vi "Begin Initialization.vi"   [LabVIEW 2016]
uses:
  <vilib>/Rock Robotics/WPI/DriverStation/WPI_DriverStationRobotMode2.ctl
  <vilib>/Rock Robotics/WPI/Joystick/WPI_JoystickDeviceEnum.ctl
  <vilib>/Rock Robotics/WPI/ThirdParty/CanMotor/TalonSRX/WPI_CANTalonSRX_APIControlMode.ctl
  <vilib>/Rock Robotics/WPI/Solenoid/WPI_SolenoidChannel.ctl
  <vilib>/Rock Robotics/SystemInterfaces/DIO/FPGA_DIOChannel.ctl
  <vilib>/Rock Robotics/WPI/ThirdParty/CanMotor/TalonSRX/WPI_CANTalonSRX_APIFeedbackSelect.ctl
  <vilib>/Rock Robotics/WPI/Solenoid/WPI_SolenoidValue.ctl
  <vilib>/Rock Robotics/SystemInterfaces/DIO/FPGA_DIOPWMChannel.ctl
  Robot Global Data.vi
  <vilib>/Rock Robotics/WPI/Solenoid/WPI_SolenoidOpenDouble.vi
  Global Variables/Robot Status.vi
  <vilib>/Rock Robotics/WPI/MotorControl/WPI_MotorControlOpen Talon.vi
  Global Variables/Refnum Names.vi
  <vilib>/Rock Robotics/WPI/ThirdParty/Sensors/Pigeon IMU/CTRE_PigeonIMU_Open_TalonSRX.vi
  <vilib>/Rock Robotics/WPI/Solenoid/WPI_SolenoidSetEnum.vi
  Global Variables/Folder Names.vi
  Global Variables/MotionProfile.vi
  Global Variables/Low Gear Calibrations.vi
  Global Variables/High Gear Calibrations.vi
types:
  T1 = typedef "WPI_CANTalonSRX_APIControlMode.ctl" = enum8{"Percent VBus", "Speed", "Position", "Slave", "Unchanged / Invalid", "Voltage Compensation", "Current", "Motion Profile", "Motion Magic"}
  T2 = typedef "FPGA_DIOChannel.ctl" = enum8{"DIO 0", "DIO 1", "DIO 2", "DIO 3", "DIO 4", "DIO 5", "DIO 6", "DIO 7", "DIO 8", "DIO 9", "DIO MXP 0", "DIO MXP 1", "DIO MXP 2", "DIO MXP 3", "DIO MXP 4", "DIO MXP 5", "DIO MXP 6", "DIO MXP 7", "DIO MXP 8", "DIO MXP 9", "DIO MXP 10", "DIO MXP 11", "DIO MXP 12", "DIO MXP 13", "DIO MXP 14", "DIO MXP 15", "SPI Port CS1", "SPI Port CS2", "SPI Port CS3", "SPI Port MISO", "SPI Port MOSI", "Invalid"}
  T3 = typedef "WPI_SolenoidValue.ctl" = enum16{"Off", "On", "Forward", "Reverse"}
  T4 = typedef "WPI_SolenoidChannel.ctl" = enum8{"Solenoid 0", "Solenoid 1", "Solenoid 2", "Solenoid 3", "Solenoid 4", "Solenoid 5", "Solenoid 6", "Solenoid 7", "Invalid"}
  T5 = typedef "FPGA_DIOPWMChannel.ctl" = enum8{"PWM 0", "PWM 1", "PWM 2", "PWM 3", "PWM 4", "PWM 5", "PWM 6", "PWM 7", "PWM 8", "PWM 9", "PWM MXP 0", "PWM MXP 1", "PWM MXP 2", "PWM MXP 3", "PWM MXP 4", "PWM MXP 5", "PWM MXP 6", "PWM MXP 7", "PWM MXP 8", "PWM MXP 9", "Invalid"}
  T6 = typedef "WPI_JoystickDeviceEnum.ctl" = enum16{"USB 0", "USB 1", "USB 2", "USB 3", "USB 4", "USB 5"}
  T7 = typedef "WPI_CANTalonSRX_APIFeedbackSelect.ctl" = enum16{"Digital Quadrature Encoder", "Analog Potentiometer", "Analog Encoder", "Count on Quad-A (Rising-Edge)", "Count on Quad-A (Falling-Edge)", "CTR Magnetic Enc (Absolute)", "CTR Magnetic Enc (Relative)", "Pulse Width"}
  T8 = typedef "WPI_DriverStationRobotMode2.ctl" = enum16{"Autonomous Disabled", "Autonomous Enabled", "Teleop Disabled", "Teleop Enabled", "Disconnected", "Finish", "Test Disabled", "Test Enabled", "Emergency Stopped"}
  T9 = typedef "WPI_JoystickDevRef.ctl" = cluster{"Device":T6}
  T10 = typedef "WPI_MotorControlDeviceRef.ctl" = cluster{"DeviceStatus":errorcluster, "Type":T11, "PWM":cluster{"PWM Channel":T5, "DeadBand":T12}, "CAN":cluster{"Device Number":u8, "SetOutput VI Ref":variant, "GetOutput VI Ref":variant, "Enable VI Ref":variant, "Disable VI Ref":variant, "Data":variant}, "Invert":bool}
  T11 = typedef "WPI_MotorControlType.ctl" = enum16{"PWM", "CAN"}
  T12 = typedef "WPI_PWMDeadband.ctl" = cluster{"Name":string, "maxPositivePwm":i32, "minPositivePwm":i32, "centerPwm":i32, "maxNegativePwm":i32, "minNegativePwm":i32, "angularRange":u16}
  T13 = typedef "MotionProfile TypeDef.ctl" = cluster{"Left MP Array":dbl[][], "Left MP Index":dbl, "Semaphore":bool, "Right MP Array":dbl[][], "Right MP Index":dbl}
  T14 = typedef "CTRE_PigeonIMU_DeviceRef.ctl" = cluster{"DeviceStatus":errorcluster, "Device Number":u8, "Type":T15, "Device ID":u32}
  T15 = typedef "CTRE_PigeonIMU_ConnectionType.ctl" = u32
  T16 = typedef "WPI_SolenoidDevRef.ctl" = cluster{"DevStatus":errorcluster, "Pneumatics Control Module":u8, "Forward Solenoid Channel":T4, "Reverse Solenoid Channel":T4}
  T17 = typedef "WPI_DigitalOutputDevRef.ctl" = cluster{"DIO Channel":T2, "DevStatus":errorcluster}
  T18 = typedef "WPI_DigitalInputDevRef.ctl" = cluster{"DevStatus":errorcluster, "DIO Channel":T2}
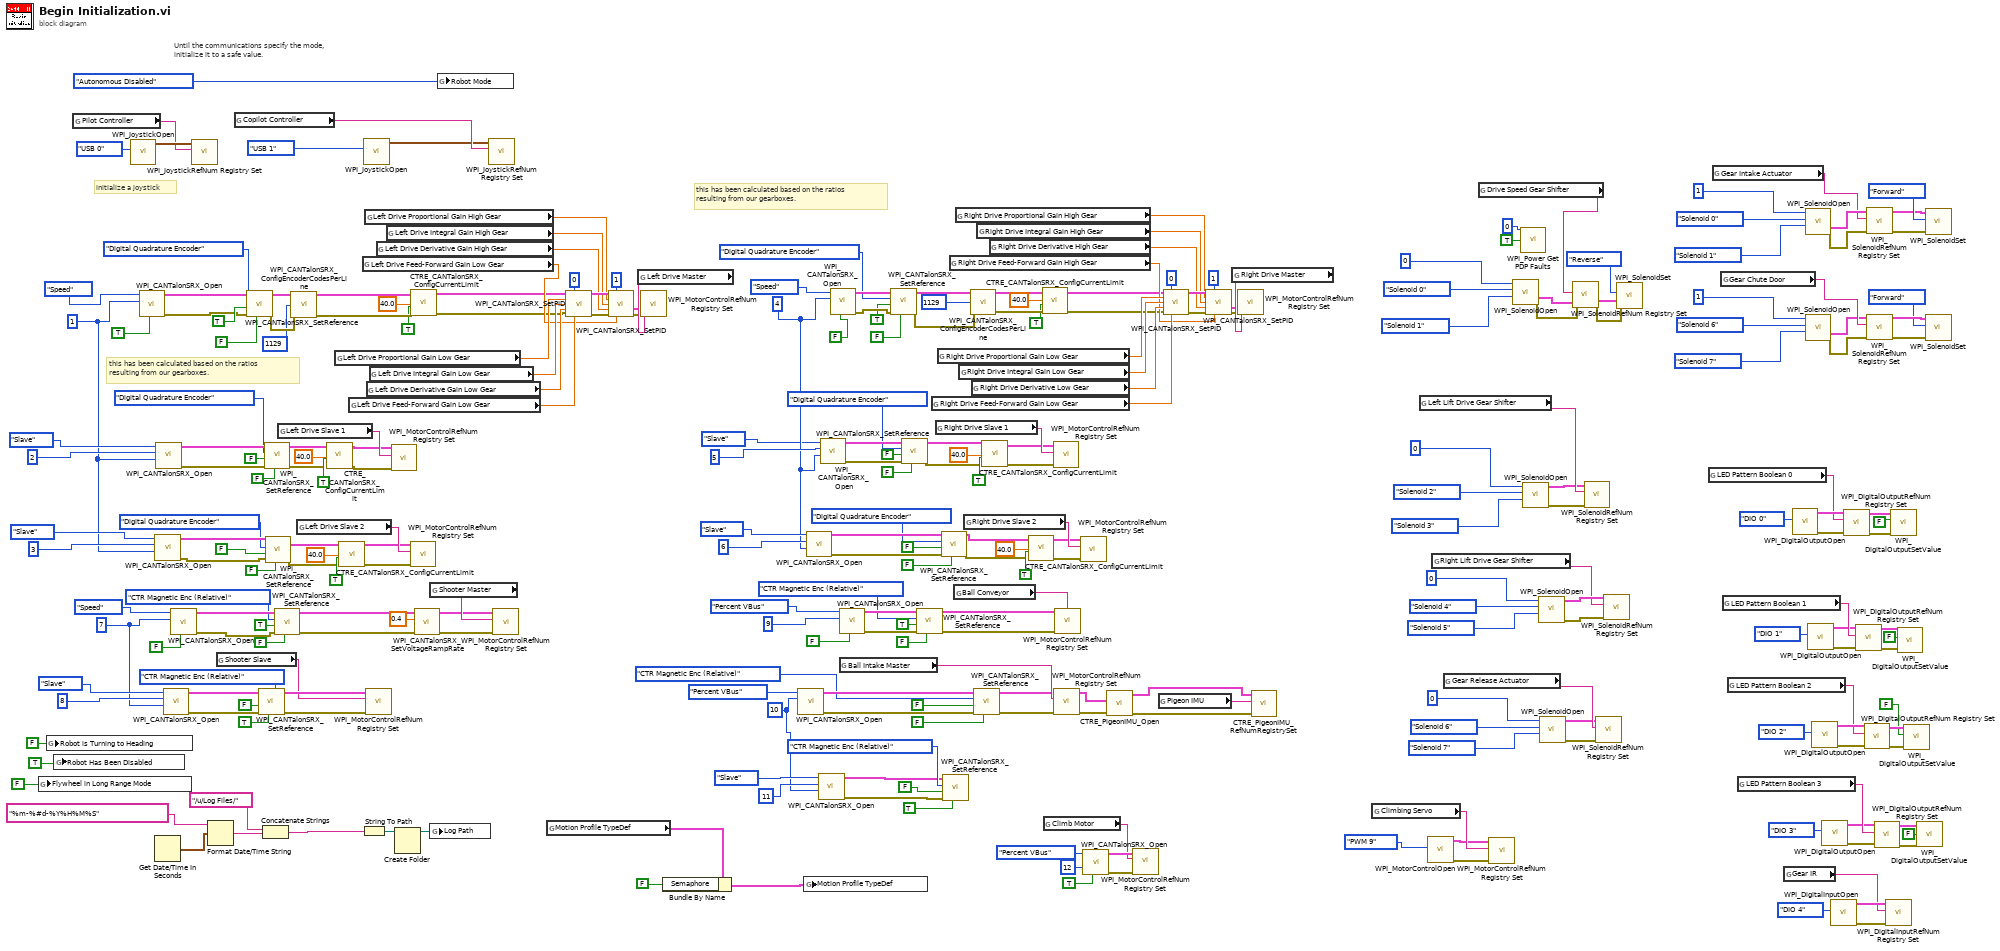
[diagram p0: block diagram]
diagram:
  w155 = u8 10 ("Device Number")
  w259 = u8 7 ("Device Number")
  w258 = u8 4 ("Device Number")
  w260 = u8 1 ("Device Number")
  # "this has been calculated based on the ratios\nresulting from our gearboxes."
  # "this has been calculated based on the ratios\nresulting from our gearboxes."
  # "initialize a joystick"
  # "Until the communications specify the mode,\ninitialize it to a safe value."
  n1 = global write "Robot Status.vi" "Flywheel in Long Range Mode"(FALSE) -> ()
  n2 = global write "Robot Status.vi" "Robot is Turning to Heading"(FALSE ("Robot is Turning to Heading")) -> ()
  n3 = global write "Robot Status.vi" "Robot Has Been Disabled"(TRUE) -> ()
  n4 = global read "Refnum Names.vi" "Pilot Controller"() -> (w248:string)
  n5 = call <vilib>:"WPI_JoystickOpen.vi"("JoystickDevice"=WPI_JoystickDeviceEnum."USB 0") -> ("JoystickDevRef"=w283:T9)  [unwired: 10 in]
  n6 = call <vilib>:"WPI_CANTalonSRX_Open.vi"("Invert"=TRUE, "Device Number"=w260, "Control Mode"=WPI_CANTalonSRX_APIControlMode."Speed") -> ("error out"=w195:errorcluster, "CAN Talon SRX Ref"=w280:T10)  [unwired: 7 in]
  n7 = call <vilib>:"WPI_CANTalonSRX_Open.vi"("Master Device Number"=w260, "Device Number"=u8 3, "Control Mode"=WPI_CANTalonSRX_APIControlMode."Slave") -> ("error out"=w193:errorcluster, "CAN Talon SRX Ref"=w273:T10)  [unwired: 7 in]
  n8 = Get Date/Time In Seconds() -> (seconds since 1Jan1904=w137:timestamp)
  n9 = call <vilib>:"WPI_CANTalonSRX_Open.vi"("Master Device Number"=w260, "Device Number"=u8 2, "Control Mode"=WPI_CANTalonSRX_APIControlMode."Slave") -> ("error out"=w194:errorcluster, "CAN Talon SRX Ref"=w278:T10)  [unwired: 7 in]
  n10 = call <vilib>:"WPI_CANTalonSRX_Open.vi"("Master Device Number"=w259, "Device Number"=u8 8, "Control Mode"=WPI_CANTalonSRX_APIControlMode."Slave") -> ("error out"=w187:errorcluster, "CAN Talon SRX Ref"=w261:T10)  [unwired: 7 in]
  n11 = call <vilib>:"WPI_CANTalonSRX_Open.vi"("Invert"=FALSE, "Device Number"=w259, "Control Mode"=WPI_CANTalonSRX_APIControlMode."Speed") -> ("error out"=w189:errorcluster, "CAN Talon SRX Ref"=w265:T10)  [unwired: 7 in]
  n12 = call <vilib>:"WPI_JoystickRefNum Registry Set.vi"("refnum name"=w248, "JoystickDevRef"=w283) -> ()  [unwired: 8 in, 2 out]
  n13 = Format Date/Time String(time format string (%c)="%m-%#d-%Y%H%M%S", seconds (now)=w137) -> (date/time string=w135:string)  [unwired: 1 in]
  n14 = global read "Refnum Names.vi" "Shooter Slave"() -> (w123:string)
  n15 = global read "Refnum Names.vi" "Copilot Controller"() -> (w153:string)
  n16 = call <vilib>:"WPI_CANTalonSRX_SetReference.vi"("Reverse Closed-Loop Output"=FALSE, "error in (no error)"=w195, "Reverse Feedback Sensor"=TRUE, "Feedback Reference"=WPI_CANTalonSRX_APIFeedbackSelect."Digital Quadrature Encoder", "CAN Talon SRX Ref"=w280) -> ("error out"=w150:errorcluster, "CAN Talon SRX Ref"=w204:T10)  [unwired: 5 in]
  n17 = call <vilib>:"WPI_CANTalonSRX_SetReference.vi"("Reverse Closed-Loop Output"=TRUE, "error in (no error)"=w187, "Reverse Feedback Sensor"=FALSE, "Feedback Reference"=WPI_CANTalonSRX_APIFeedbackSelect."CTR Magnetic Enc (Relative)", "CAN Talon SRX Ref"=w261) -> ("error out"=w125:errorcluster, "CAN Talon SRX Ref"=w124:T10)  [unwired: 5 in]
  n18 = Concatenate Strings("/u/Log Files/" ("string"), w135) -> (w133:string)
  n19 = call <vilib>:"WPI_CANTalonSRX_SetReference.vi"("Reverse Closed-Loop Output"=FALSE, "error in (no error)"=w194, "Reverse Feedback Sensor"=FALSE, "Feedback Reference"=WPI_CANTalonSRX_APIFeedbackSelect."Digital Quadrature Encoder", "CAN Talon SRX Ref"=w278) -> ("error out"=w19:errorcluster, "CAN Talon SRX Ref"=w20:T10)  [unwired: 5 in]
  n20 = call <vilib>:"WPI_CANTalonSRX_SetReference.vi"("Reverse Closed-Loop Output"=FALSE, "error in (no error)"=w193, "Reverse Feedback Sensor"=FALSE, "Feedback Reference"=WPI_CANTalonSRX_APIFeedbackSelect."Digital Quadrature Encoder", "CAN Talon SRX Ref"=w273) -> ("error out"=w14:errorcluster, "CAN Talon SRX Ref"=w15:T10)  [unwired: 5 in]
  n21 = call <vilib>:"WPI_CANTalonSRX_SetReference.vi"("Reverse Closed-Loop Output"=FALSE, "error in (no error)"=w189, "Reverse Feedback Sensor"=TRUE, "Feedback Reference"=WPI_CANTalonSRX_APIFeedbackSelect."CTR Magnetic Enc (Relative)", "CAN Talon SRX Ref"=w265) -> ("error out"=w120:errorcluster, "CAN Talon SRX Ref"=w122:T10)  [unwired: 5 in]
  n22 = global read "Refnum Names.vi" "Left Drive Slave 1"() -> (w50:string)
  n23 = call <vilib>:"WPI_CANTalonSRX_ConfigEncoderCodesPerLine.vi"("CAN Talon SRX Ref"=w204, "Number Encoder Lines\n(Counts Per Rotation)"=u32 1129 ("Number Encoder Lines\n(Counts Per Rotation)"), "error in (no error)"=w150) -> ("CAN Talon SRX Ref"=w36:T10, "error out"=w35:errorcluster)  [unwired: 11 in]
  n24 = global read "Refnum Names.vi" "Left Drive Slave 2"() -> (w49:string)
  n25 = call <vilib>:"CTRE_CANTalonSRX_ConfigCurrentLimit.vi"("error in (no error)"=w19, "Enable Current Limit?"=TRUE, "Current Limit (Amps)"=40.0, "CAN Talon SRX Ref"=w20) -> ("error out"=w21:errorcluster, "CAN Talon SRX Ref"=w22:T10)  [unwired: 6 in]
  n26 = global read "Low Gear Calibrations.vi" "Left Drive Proportional Gain Low Gear"() -> (w111:dbl)
  n27 = call <vilib>:"CTRE_CANTalonSRX_ConfigCurrentLimit.vi"("error in (no error)"=w14, "Enable Current Limit?"=TRUE, "Current Limit (Amps)"=40.0, "CAN Talon SRX Ref"=w15) -> ("error out"=w13:errorcluster, "CAN Talon SRX Ref"=w16:T10)  [unwired: 6 in]
  n28 = global read "Low Gear Calibrations.vi" "Left Drive Feed-Forward Gain Low Gear"() -> (w108:dbl)
  n29 = String To Path(string=w133) -> (path=w132:path)
  n30 = global read "High Gear Calibrations.vi" "Left Drive Feed-Forward Gain Low Gear"() -> (w67:dbl)
  n31 = call <vilib>:"WPI_JoystickOpen.vi"("JoystickDevice"=WPI_JoystickDeviceEnum."USB 1") -> ("JoystickDevRef"=w151:T9)  [unwired: 10 in]
  n32 = global read "High Gear Calibrations.vi" "Left Drive Proportional Gain High Gear"() -> (w105:dbl)
  n33 = call <vilib>:"WPI_MotorControlRefNum Registry Set.vi"("error in (no error)"=w125, "refnum name"=w123, "MotorControlDevRef"=w124) -> ()  [unwired: 7 in, 2 out]
  n34 = global read "Low Gear Calibrations.vi" "Left Drive Derivative Gain Low Gear"() -> (w109:dbl)
  n35 = global read "Low Gear Calibrations.vi" "Left Drive Integral Gain Low Gear"() -> (w110:dbl)
  n36 = global read "High Gear Calibrations.vi" "Left Drive Derivative Gain High Gear"() -> (w107:dbl)
  n37 = global read "High Gear Calibrations.vi" "Left Drive Integral Gain High Gear"() -> (w106:dbl)
  n38 = call <vilib>:"WPI_MotorControlRefNum Registry Set.vi"("error in (no error)"=w21, "refnum name"=w50, "MotorControlDevRef"=w22) -> ()  [unwired: 7 in, 2 out]
  n39 = Create Folder(path (use dialog)=w132) -> (created path=w131:path)  [unwired: 2 in, 2 out]
  n40 = call <vilib>:"WPI_MotorControlRefNum Registry Set.vi"("error in (no error)"=w13, "refnum name"=w49, "MotorControlDevRef"=w16) -> ()  [unwired: 7 in, 2 out]
  n41 = call <vilib>:"CTRE_CANTalonSRX_ConfigCurrentLimit.vi"("error in (no error)"=w35, "Enable Current Limit?"=TRUE, "Current Limit (Amps)"=40.0, "CAN Talon SRX Ref"=w36) -> ("error out"=w34:errorcluster, "CAN Talon SRX Ref"=w33:T10)  [unwired: 6 in]
  n42 = call <vilib>:"WPI_CANTalonSRX_SetVoltageRampRate.vi"("error in (no error)"=w120, "Throttle Ramp Rate (percent/s)"=0.4, "CAN Talon SRX Ref"=w122) -> ("error out"=w119:errorcluster, "CAN Talon SRX Ref"=w121:T10)  [unwired: 7 in]
  n43 = global read "Refnum Names.vi" "Shooter Master"() -> (w266:string)
  n44 = global write "Folder Names.vi" "Log Path"(w131) -> ()
  n45 = global write "Robot Global Data.vi" "Robot Mode"(WPI_DriverStationRobotMode2."Autonomous Disabled" ("Robot Mode")) -> ()
  n46 = call <vilib>:"WPI_JoystickRefNum Registry Set.vi"("refnum name"=w153, "JoystickDevRef"=w151) -> ()  [unwired: 8 in, 2 out]
  n47 = call <vilib>:"WPI_MotorControlRefNum Registry Set.vi"("error in (no error)"=w119, "refnum name"=w266, "MotorControlDevRef"=w121) -> ()  [unwired: 7 in, 2 out]
  n48 = global read "MotionProfile.vi" "Motion Profile TypeDef"() -> (w74:T13)
  n49 = call <vilib>:"WPI_CANTalonSRX_SetPID.vi"("CAN Talon SRX Ref"=w33, "Parameter Slot"=u8 0, "P"=w111, "I"=w110, "D"=w109, "error in (no error)"=w34, "F"=w108) -> ("CAN Talon SRX Ref"=w114:T10, "error out"=w115:errorcluster)  [unwired: 7 in]
  n50 = call <vilib>:"WPI_CANTalonSRX_SetPID.vi"("CAN Talon SRX Ref"=w114, "Parameter Slot"=u8 1, "P"=w105, "I"=w106, "D"=w107, "error in (no error)"=w115, "F"=w67) -> ("CAN Talon SRX Ref"=w117:T10, "error out"=w116:errorcluster)  [unwired: 7 in]
  n51 = global read "Refnum Names.vi" "Left Drive Master"() -> (w279:string)
  n52 = call <vilib>:"WPI_MotorControlRefNum Registry Set.vi"("error in (no error)"=w116, "refnum name"=w279, "MotorControlDevRef"=w117) -> ()  [unwired: 7 in, 2 out]
  n53 = Bundle By Name(cluster=w74, "Semaphore"=FALSE) -> (w72:T13)
  n54 = call <vilib>:"WPI_CANTalonSRX_Open.vi"("Device Number"=w155, "Control Mode"=WPI_CANTalonSRX_APIControlMode."Percent VBus") -> ("error out"=w254:errorcluster, "CAN Talon SRX Ref"=w255:T10)  [unwired: 8 in]
  n55 = global write "MotionProfile.vi" "Motion Profile TypeDef"(w72) -> ()
  n56 = call <vilib>:"WPI_CANTalonSRX_Open.vi"("Master Device Number"=w258, "Device Number"=u8 6, "Control Mode"=WPI_CANTalonSRX_APIControlMode."Slave") -> ("error out"=w175:errorcluster, "CAN Talon SRX Ref"=w174:T10)  [unwired: 7 in]
  n57 = call <vilib>:"WPI_CANTalonSRX_Open.vi"("Master Device Number"=w155, "Device Number"=u8 11, "Control Mode"=WPI_CANTalonSRX_APIControlMode."Slave") -> ("error out"=w154:errorcluster, "CAN Talon SRX Ref"=w156:T10)  [unwired: 7 in]
  n58 = call <vilib>:"WPI_CANTalonSRX_Open.vi"("Master Device Number"=w258, "Device Number"=u8 5, "Control Mode"=WPI_CANTalonSRX_APIControlMode."Slave") -> ("error out"=w179:errorcluster, "CAN Talon SRX Ref"=w269:T10)  [unwired: 7 in]
  n59 = call <vilib>:"WPI_CANTalonSRX_Open.vi"("Invert"=FALSE, "Device Number"=w258, "Control Mode"=WPI_CANTalonSRX_APIControlMode."Speed") -> ("error out"=w183:errorcluster, "CAN Talon SRX Ref"=w272:T10)  [unwired: 7 in]
  n60 = call <vilib>:"WPI_CANTalonSRX_Open.vi"("Invert"=FALSE, "Device Number"=u8 9, "Control Mode"=WPI_CANTalonSRX_APIControlMode."Percent VBus") -> ("error out"=w251:errorcluster, "CAN Talon SRX Ref"=w250:T10)  [unwired: 7 in]
  n61 = global read "Refnum Names.vi" "Ball Intake Master"() -> (w256:string)
  n62 = call <vilib>:"WPI_CANTalonSRX_SetReference.vi"("Reverse Closed-Loop Output"=FALSE, "error in (no error)"=w183, "Reverse Feedback Sensor"=TRUE, "Feedback Reference"=WPI_CANTalonSRX_APIFeedbackSelect."Digital Quadrature Encoder", "CAN Talon SRX Ref"=w272) -> ("error out"=w148:errorcluster, "CAN Talon SRX Ref"=w184:T10)  [unwired: 5 in]
  n63 = call <vilib>:"WPI_CANTalonSRX_SetReference.vi"("Reverse Closed-Loop Output"=FALSE, "error in (no error)"=w179, "Reverse Feedback Sensor"=FALSE, "Feedback Reference"=WPI_CANTalonSRX_APIFeedbackSelect."Digital Quadrature Encoder", "CAN Talon SRX Ref"=w269) -> ("error out"=w8:errorcluster, "CAN Talon SRX Ref"=w9:T10)  [unwired: 5 in]
  n64 = call <vilib>:"WPI_CANTalonSRX_SetReference.vi"("Reverse Closed-Loop Output"=FALSE, "Reverse Feedback Sensor"=TRUE, "Feedback Reference"=WPI_CANTalonSRX_APIFeedbackSelect."CTR Magnetic Enc (Relative)", "CAN Talon SRX Ref"=w250) -> ("CAN Talon SRX Ref"=w170:T10)  [unwired: 6 in, 1 out]
  n65 = global read "Low Gear Calibrations.vi" "Right Drive Feed-Forward Gain Low Gear"() -> (w94:dbl)
  n66 = global read "Refnum Names.vi" "Right Drive Slave 1"() -> (w48:string)
  n67 = global read "Low Gear Calibrations.vi" "Right Drive Proportional Gain Low Gear"() -> (w97:dbl)
  n68 = call <vilib>:"WPI_CANTalonSRX_SetReference.vi"("Reverse Closed-Loop Output"=FALSE, "error in (no error)"=w175, "Reverse Feedback Sensor"=FALSE, "Feedback Reference"=WPI_CANTalonSRX_APIFeedbackSelect."Digital Quadrature Encoder", "CAN Talon SRX Ref"=w174) -> ("error out"=w2:errorcluster, "CAN Talon SRX Ref"=w3:T10)  [unwired: 5 in]
  n69 = call <vilib>:"WPI_CANTalonSRX_SetReference.vi"("Reverse Closed-Loop Output"=TRUE, "error in (no error)"=w154, "Reverse Feedback Sensor"=FALSE, "Feedback Reference"=WPI_CANTalonSRX_APIFeedbackSelect."CTR Magnetic Enc (Relative)", "CAN Talon SRX Ref"=w156) -> ()  [unwired: 5 in, 2 out]
  n70 = global read "High Gear Calibrations.vi" "Right Drive Feed-Forward Gain High Gear"() -> (w68:dbl)
  n71 = global read "Refnum Names.vi" "Ball Conveyor"() -> (w249:string)
  n72 = global read "High Gear Calibrations.vi" "Right Drive Proportional Gain High Gear"() -> (w91:dbl)
  n73 = global read "Low Gear Calibrations.vi" "Right Drive Integral Gain Low Gear"() -> (w96:dbl)
  n74 = global read "Refnum Names.vi" "Right Drive Slave 2"() -> (w47:string)
  n75 = call <vilib>:"WPI_CANTalonSRX_ConfigEncoderCodesPerLine.vi"("CAN Talon SRX Ref"=w184, "Number Encoder Lines\n(Counts Per Rotation)"=u32 1129 ("Number Encoder Lines\n(Counts Per Rotation)"), "error in (no error)"=w148) -> ("CAN Talon SRX Ref"=w32:T10, "error out"=w31:errorcluster)  [unwired: 11 in]
  n76 = global read "Low Gear Calibrations.vi" "Right Drive Derivative Low Gear"() -> (w95:dbl)
  n77 = call <vilib>:"WPI_CANTalonSRX_SetReference.vi"("Reverse Closed-Loop Output"=FALSE, "Reverse Feedback Sensor"=FALSE, "Feedback Reference"=WPI_CANTalonSRX_APIFeedbackSelect."CTR Magnetic Enc (Relative)", "CAN Talon SRX Ref"=w255) -> ("CAN Talon SRX Ref"=w165:T10)  [unwired: 6 in, 1 out]
  n78 = global read "High Gear Calibrations.vi" "Right Drive Integral Gain High Gear"() -> (w92:dbl)
  n79 = call <vilib>:"CTRE_CANTalonSRX_ConfigCurrentLimit.vi"("error in (no error)"=w8, "Enable Current Limit?"=TRUE, "Current Limit (Amps)"=40.0, "CAN Talon SRX Ref"=w9) -> ("error out"=w7:errorcluster, "CAN Talon SRX Ref"=w10:T10)  [unwired: 6 in]
  n80 = global read "High Gear Calibrations.vi" "Right Drive Derivative High Gear"() -> (w93:dbl)
  n81 = call <vilib>:"CTRE_CANTalonSRX_ConfigCurrentLimit.vi"("error in (no error)"=w2, "Enable Current Limit?"=TRUE, "Current Limit (Amps)"=40.0, "CAN Talon SRX Ref"=w3) -> ("error out"=w1:errorcluster, "CAN Talon SRX Ref"=w4:T10)  [unwired: 6 in]
  n82 = call <vilib>:"CTRE_CANTalonSRX_ConfigCurrentLimit.vi"("error in (no error)"=w31, "Enable Current Limit?"=TRUE, "Current Limit (Amps)"=40.0, "CAN Talon SRX Ref"=w32) -> ("error out"=w30:errorcluster, "CAN Talon SRX Ref"=w29:T10)  [unwired: 6 in]
  n83 = global read "Refnum Names.vi" "Climb Motor"() -> (w38:string)
  n84 = call <vilib>:"WPI_MotorControlRefNum Registry Set.vi"("error in (no error)"=w7, "refnum name"=w48, "MotorControlDevRef"=w10) -> ()  [unwired: 7 in, 2 out]
  n85 = call <vilib>:"WPI_MotorControlRefNum Registry Set.vi"("error in (no error)"=w254, "refnum name"=w256, "MotorControlDevRef"=w165) -> ("error out"=w51:errorcluster, "MotorControlDevRef"=w52:T10)  [unwired: 7 in]
  n86 = call <vilib>:"WPI_MotorControlRefNum Registry Set.vi"("error in (no error)"=w251, "refnum name"=w249, "MotorControlDevRef"=w170) -> ()  [unwired: 7 in, 2 out]
  n87 = call <vilib>:"WPI_MotorControlRefNum Registry Set.vi"("error in (no error)"=w1, "refnum name"=w47, "MotorControlDevRef"=w4) -> ()  [unwired: 7 in, 2 out]
  n88 = call <vilib>:"WPI_CANTalonSRX_Open.vi"("Invert"=TRUE, "Device Number"=u8 12, "Control Mode"=WPI_CANTalonSRX_APIControlMode."Percent VBus") -> ("error out"=w41:errorcluster, "CAN Talon SRX Ref"=w42:T10)  [unwired: 7 in]
  n89 = call-poly <vilib>:"CTRE_PigeonIMU_Open.vi"("error in"=w51, "CAN Talon SRX Ref"=w52) -> ("error out"=w53:errorcluster, "PigeonIMUDevRef"=w55:T14)  [unwired: 8 in]
  n90 = call <vilib>:"WPI_MotorControlRefNum Registry Set.vi"("error in (no error)"=w41, "refnum name"=w38, "MotorControlDevRef"=w42) -> ()  [unwired: 7 in, 2 out]
  n91 = global read "Refnum Names.vi" "Pigeon IMU"() -> (w54:string)
  n92 = call <vilib>:"WPI_CANTalonSRX_SetPID.vi"("CAN Talon SRX Ref"=w29, "Parameter Slot"=u8 0, "P"=w97, "I"=w96, "D"=w95, "error in (no error)"=w30, "F"=w94) -> ("CAN Talon SRX Ref"=w100:T10, "error out"=w101:errorcluster)  [unwired: 7 in]
  n93 = call <vilib>:"WPI_CANTalonSRX_SetPID.vi"("CAN Talon SRX Ref"=w100, "Parameter Slot"=u8 1, "P"=w91, "I"=w92, "D"=w93, "error in (no error)"=w101, "F"=w68) -> ("CAN Talon SRX Ref"=w103:T10, "error out"=w102:errorcluster)  [unwired: 7 in]
  n94 = global read "Refnum Names.vi" "Right Drive Master"() -> (w104:string)
  n95 = call <vilib>:"WPI_MotorControlRefNum Registry Set.vi"("error in (no error)"=w102, "refnum name"=w104, "MotorControlDevRef"=w103) -> ()  [unwired: 7 in, 2 out]
  n96 = call <vilib>:"CTRE_PigeonIMU_RefNumRegistrySet.vi"("error in (no error)"=w53, "refnum name"=w54, "PigeonIMUDevRef"=w55) -> ()  [unwired: 7 in, 2 out]
  n97 = global read "Refnum Names.vi" "Climbing Servo"() -> (w130:string)
  n98 = global read "Refnum Names.vi" "Left Lift Drive Gear Shifter"() -> (w244:string)
  n99 = call-poly <vilib>:"WPI_MotorControlOpen.vi"("PWM Channel"=FPGA_DIOPWMChannel."PWM 9") -> ("error out"=w129:errorcluster, "MotorControlDeviceRef"=w127:T10)  [unwired: 9 in]
  n100 = global read "Refnum Names.vi" "Right Lift Drive Gear Shifter"() -> (w233:string)
  n101 = global read "Refnum Names.vi" "Gear Release Actuator"() -> (w232:string)
  n102 = global read "Refnum Names.vi" "Drive Speed Gear Shifter"() -> (w245:string)
  n103 = call <vilib>:"WPI_MotorControlRefNum Registry Set.vi"("error in (no error)"=w129, "refnum name"=w130, "MotorControlDevRef"=w127) -> ()  [unwired: 7 in, 2 out]
  n104 = call-poly <vilib>:"WPI_SolenoidOpen.vi"("Reverse Solenoid Channel"=WPI_SolenoidChannel."Solenoid 1", "Forward Solenoid Channel"=WPI_SolenoidChannel."Solenoid 0", "Pneumatics Control Module (0)"=u8 0) -> ("error out"=w140:errorcluster, "SolenoidDevRef"=w146:T16)  [unwired: 7 in]
  n105 = call <vilib>:"WPI_Power Get PDP Faults.vi"("Power Distribution Panel (0)"=u8 0, "Clear Sticky Faults"=TRUE) -> ()  [unwired: 9 in, 5 out]
  n106 = call-poly <vilib>:"WPI_SolenoidOpen.vi"("Reverse Solenoid Channel"=WPI_SolenoidChannel."Solenoid 3", "Forward Solenoid Channel"=WPI_SolenoidChannel."Solenoid 2", "Pneumatics Control Module (0)"=u8 0) -> ("error out"=w239:errorcluster, "SolenoidDevRef"=w240:T16)  [unwired: 7 in]
  n107 = call-poly <vilib>:"WPI_SolenoidOpen.vi"("Reverse Solenoid Channel"=WPI_SolenoidChannel."Solenoid 5", "Forward Solenoid Channel"=WPI_SolenoidChannel."Solenoid 4", "Pneumatics Control Module (0)"=u8 0) -> ("error out"=w238:errorcluster, "SolenoidDevRef"=w237:T16)  [unwired: 7 in]
  n108 = call-poly <vilib>:"WPI_SolenoidOpen.vi"("Reverse Solenoid Channel"=WPI_SolenoidChannel."Solenoid 7", "Forward Solenoid Channel"=WPI_SolenoidChannel."Solenoid 6", "Pneumatics Control Module (0)"=u8 0) -> ("error out"=w227:errorcluster, "SolenoidDevRef"=w228:T16)  [unwired: 7 in]
  n109 = call <vilib>:"WPI_SolenoidRefNum Registry Set.vi"("error in (no error)"=w140, "refnum name"=w245, "SolenoidDevRef"=w146) -> ("error out"=w142:errorcluster, "SolenoidDevRef"=w141:T16)  [unwired: 7 in]
  n110 = call <vilib>:"WPI_SolenoidRefNum Registry Set.vi"("error in (no error)"=w239, "refnum name"=w244, "SolenoidDevRef"=w240) -> ()  [unwired: 7 in, 2 out]
  n111 = call <vilib>:"WPI_SolenoidRefNum Registry Set.vi"("error in (no error)"=w227, "refnum name"=w232, "SolenoidDevRef"=w228) -> ()  [unwired: 7 in, 2 out]
  n112 = call <vilib>:"WPI_SolenoidRefNum Registry Set.vi"("error in (no error)"=w238, "refnum name"=w233, "SolenoidDevRef"=w237) -> ()  [unwired: 7 in, 2 out]
  n113 = call-poly <vilib>:"WPI_SolenoidSet.vi"("error in (no error)"=w142, "Value"=WPI_SolenoidValue."Reverse", "SolenoidDevRef"=w141) -> ()  [unwired: 7 in, 2 out]
  n114 = global read "Refnum Names.vi" "LED Pattern Boolean 0"() -> (w218:string)
  n115 = global read "Refnum Names.vi" "Gear Intake Actuator"() -> (w221:string)
  n116 = global read "Refnum Names.vi" "Gear Chute Door"() -> (w63:string)
  n117 = global read "Refnum Names.vi" "LED Pattern Boolean 1"() -> (w217:string)
  n118 = global read "Refnum Names.vi" "LED Pattern Boolean 2"() -> (w212:string)
  n119 = global read "Refnum Names.vi" "LED Pattern Boolean 3"() -> (w89:string)
  n120 = global read "Refnum Names.vi" "Gear IR"() -> (w43:string)
  n121 = call <vilib>:"WPI_DigitalOutputOpen.vi"("DIO Channel"=FPGA_DIOChannel."DIO 0") -> ("error out"=w210:errorcluster, "DigitalOutputDevRef"=w219:T17)  [unwired: 9 in]
  n122 = call-poly <vilib>:"WPI_SolenoidOpen.vi"("Reverse Solenoid Channel"=WPI_SolenoidChannel."Solenoid 1", "Forward Solenoid Channel"=WPI_SolenoidChannel."Solenoid 0", "Pneumatics Control Module (0)"=u8 1) -> ("error out"=w226:errorcluster, "SolenoidDevRef"=w225:T16)  [unwired: 7 in]
  n123 = call-poly <vilib>:"WPI_SolenoidOpen.vi"("Reverse Solenoid Channel"=WPI_SolenoidChannel."Solenoid 7", "Forward Solenoid Channel"=WPI_SolenoidChannel."Solenoid 6", "Pneumatics Control Module (0)"=u8 1) -> ("error out"=w58:errorcluster, "SolenoidDevRef"=w59:T16)  [unwired: 7 in]
  n124 = call <vilib>:"WPI_DigitalOutputOpen.vi"("DIO Channel"=FPGA_DIOChannel."DIO 1") -> ("error out"=w211:errorcluster, "DigitalOutputDevRef"=w216:T17)  [unwired: 9 in]
  n125 = call <vilib>:"WPI_DigitalOutputOpen.vi"("DIO Channel"=FPGA_DIOChannel."DIO 2") -> ("error out"=w209:errorcluster, "DigitalOutputDevRef"=w213:T17)  [unwired: 9 in]
  n126 = call <vilib>:"WPI_DigitalOutputOpen.vi"("DIO Channel"=FPGA_DIOChannel."DIO 3") -> ("error out"=w90:errorcluster, "DigitalOutputDevRef"=w88:T17)  [unwired: 9 in]
  n127 = call <vilib>:"WPI_DigitalInputOpen.vi"("DIO Channel"=FPGA_DIOChannel."DIO 4") -> ("error out"=w45:errorcluster, "DigitalInputDevRef"=w44:T18)  [unwired: 9 in]
  n128 = call <vilib>:"WPI_DigitalOutputRefNum Registry Set.vi"("error in (no error)"=w210, "refnum name"=w218, "DigitalOutputDevRef"=w219) -> ("error out"=w86:errorcluster, "DigitalOutputDevRef"=w85:T17)  [unwired: 7 in]
  n129 = call <vilib>:"WPI_DigitalOutputRefNum Registry Set.vi"("error in (no error)"=w211, "refnum name"=w217, "DigitalOutputDevRef"=w216) -> ("error out"=w84:errorcluster, "DigitalOutputDevRef"=w83:T17)  [unwired: 7 in]
  n130 = call <vilib>:"WPI_DigitalOutputRefNum Registry Set.vi"("error in (no error)"=w209, "refnum name"=w212, "DigitalOutputDevRef"=w213) -> ("error out"=w79:errorcluster, "DigitalOutputDevRef"=w80:T17)  [unwired: 7 in]
  n131 = call <vilib>:"WPI_SolenoidRefNum Registry Set.vi"("error in (no error)"=w226, "refnum name"=w221, "SolenoidDevRef"=w225) -> ("error out"=w69:errorcluster, "SolenoidDevRef"=w70:T16)  [unwired: 7 in]
  n132 = call <vilib>:"WPI_SolenoidRefNum Registry Set.vi"("error in (no error)"=w58, "refnum name"=w63, "SolenoidDevRef"=w59) -> ("error out"=w66:errorcluster, "SolenoidDevRef"=w65:T16)  [unwired: 7 in]
  n133 = call <vilib>:"WPI_DigitalOutputRefNum Registry Set.vi"("error in (no error)"=w90, "refnum name"=w89, "DigitalOutputDevRef"=w88) -> ("error out"=w82:errorcluster, "DigitalOutputDevRef"=w81:T17)  [unwired: 7 in]
  n134 = call <vilib>:"WPI_DigitalInputRefNum Registry Set.vi"("error in (no error)"=w45, "refnum name"=w43, "DigitalInputDevRef"=w44) -> ()  [unwired: 7 in, 2 out]
  n135 = call <vilib>:"WPI_DigitalOutputSetValue.vi"("error in (no error)"=w86, "Value"=FALSE, "DigitalOutputDevRef"=w85) -> ()  [unwired: 7 in, 2 out]
  n136 = call <vilib>:"WPI_DigitalOutputSetValue.vi"("error in (no error)"=w84, "Value"=FALSE, "DigitalOutputDevRef"=w83) -> ()  [unwired: 7 in, 2 out]
  n137 = call <vilib>:"WPI_DigitalOutputSetValue.vi"("error in (no error)"=w79, "Value"=FALSE, "DigitalOutputDevRef"=w80) -> ()  [unwired: 7 in, 2 out]
  n138 = call <vilib>:"WPI_DigitalOutputSetValue.vi"("error in (no error)"=w82, "Value"=FALSE, "DigitalOutputDevRef"=w81) -> ()  [unwired: 7 in, 2 out]
  n139 = call-poly <vilib>:"WPI_SolenoidSet.vi"("error in (no error)"=w69, "Value"=WPI_SolenoidValue."Forward", "SolenoidDevRef"=w70) -> ()  [unwired: 7 in, 2 out]
  n140 = call-poly <vilib>:"WPI_SolenoidSet.vi"("error in (no error)"=w66, "Value"=WPI_SolenoidValue."Forward", "SolenoidDevRef"=w65) -> ()  [unwired: 7 in, 2 out]
